vi "Init.vi"(5 "Stop User Event in":refnum<user-event>, 7 "Ref FP in":refnum<vi>, 8 "error in (no error)":errorcluster, 9 "Period (ms) in":i64=15, 11 "Xbox Controller in":refnum<class "Xbox Controller.lvclass">) -> (0 "error out":errorcluster, 3 "Xbox Controller out":refnum<class "Xbox Controller.lvclass">)   [LabVIEW 2024, in "Xbox Controller.lvclass"]
doc: "MIT Licence\nCopyright (c) 2024 David Grollier"
uses:
  Xbox Controller.lvclass
  Xbox Controller.lvclass/Xbox Controller.ctl
  <vilib>/Utility/error.llb/Error Cluster From Error Code.vi
  Input Device.lvclass
  <vilib>/ErrorRing/Error Ring.xnode
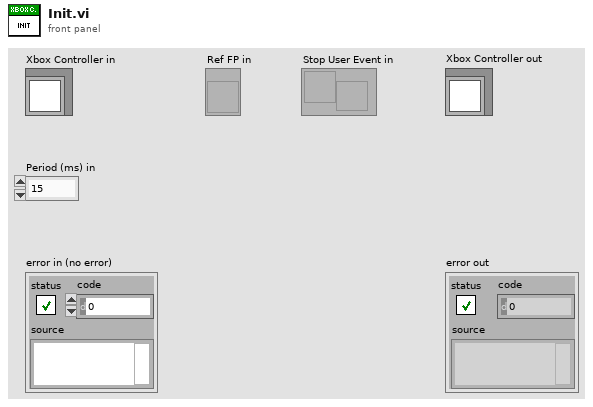
[diagram p1: front panel]
types:
  T1 = cluster{"axes total":u32, "buttons total":u32, "pov total":u32, "device name":string}[]
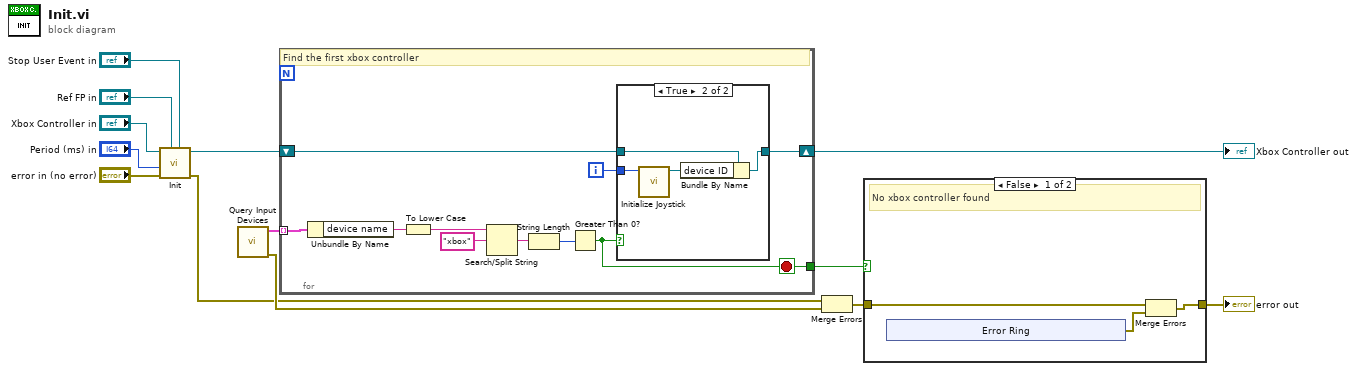
[diagram p0: block diagram]
diagram:
  n1 = call-parent "Init.vi"("Stop User Event in"="Stop User Event in", "Ref FP in"="Ref FP in", "error in (no error)"="error in (no error)", "Period (ms) in"="Period (ms) in", "Input Device in"="Xbox Controller in") -> ("error out"=w3:errorcluster, "Input Device out"=w6:refnum<class "Xbox Controller.lvclass">)  [unwired: 5 in]
  n2 = call <vilib>:"Query Input Devices.vi"() -> ("error out"=w8:errorcluster, "joystick info"=w9:T1)  [unwired: 8 in, 2 out]
  n3 = for {
    tunnel: w9 -> [w23] mode=indexing
    tunnel: [w17] -> w7
    shift-right: [w14] -> w2
    shift-left: w6 -> [w16]
    i -> [w15]
    stop <- w17 stop-if-true
    # "Find the first xbox controller"
    n4 = Unbundle By Name(w23) -> ("device name"=w18:string)
    n5 = To Lower Case(string=w18) -> (all lower case string=w22:string)
    n6 = Search/Split String(string=w22, search string/char (-)="xbox") -> (match + rest of string=w20:string)  [unwired: 1 in, 2 out]
    n7 = String Length(string=w20) -> (length=w19:i32)
    n8 = Greater Than 0?(x=w19) -> (x > 0?=w17:bool)
    n9 = case shown="True" w17 {
      tunnel: w16 -> [w24 w28]
      tunnel: w15 -> [_ w27]
      tunnel: [w24 w25] -> w14
      frame False {
      }
      frame True {
        n10 = call <vilib>:"Initialize Joystick.vi"("device index"=w27) -> ("device ID"=w26:refnum<k1>)  [unwired: 9 in, 1 out]
        n11 = Bundle By Name(cluster=w28, "device ID"=w26) -> (w25:refnum<class "Xbox Controller.lvclass">)
      }
    }
  }
  "Xbox Controller out" <- w2
  n12 = Merge Errors(w3, w8) -> (w5:errorcluster)
  n13 = case shown="False" w7 {
    tunnel: w5 -> [w31 w37]
    tunnel: [w29 w37] -> w4
    frame False {
      # "No xbox controller found"
      n14 = xnode "Error Ring"() -> ("error out"=w30:errorcluster)
      n15 = Merge Errors(w31, w30) -> (w29:errorcluster)
    }
    frame True {
      # "A xbox controller found"
    }
  }
  "error out" <- w4
